vi "Shift Zero (single).vi"(8 "error in (no error)":errorcluster, 10 "Zero x index":i32, 11 "XY-data":cluster{"X-array":dbl[], "Y-array":dbl[]}) -> (0 "error out":errorcluster, 3 "Shifted XY-data out":cluster{"X-array":dbl[], "Y-array":dbl[]} {"Y-array" format="%.2p"; "X-array" format="%.2p"})   [LabVIEW 2016, in "xy_utilities.lvlib"]
doc: "Shift the zero value of the x array by giving a new fractional x index.\n\nWire data to the data input to determine the polymorphic instance to use or manually select the instance."
uses:
  xy_utilities.lvlib
  Sort (single).vi
  <vilib>/gmath/NI_Gmath.lvlib
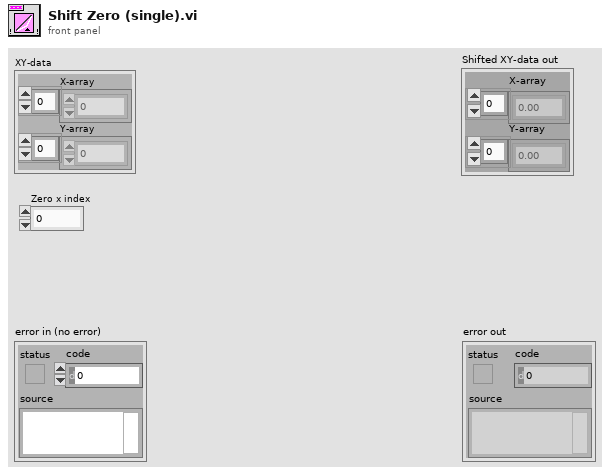
[diagram p1: front panel]
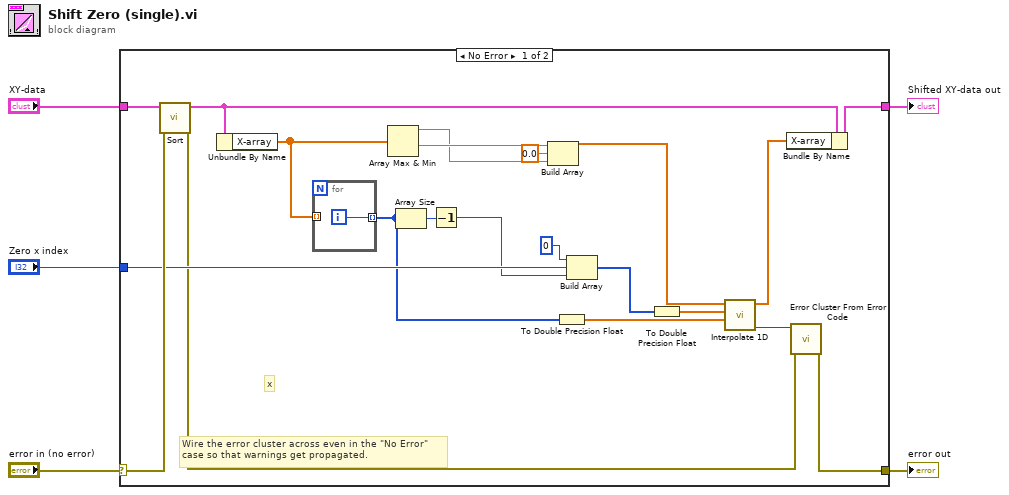
[diagram p0: block diagram]
diagram:
  n1 = case shown="No Error" "error in (no error)" {
    selector: "error in (no error)" -> [w20 w29]
    tunnel: [w8 w29] -> w4
    tunnel: "XY-data" -> [w11 w28]
    tunnel: [w26 w28] -> w2
    tunnel: "Zero x index" -> [w17 _]
    frame No Error {
      # "x"
      # "Wire the error cluster across even in the \"No Error\"\ncase so that warnings get propagated."
      n2 = call-poly "Sort.vi"("error in (no error)"=w20, "XY-data"=w11) -> ("error out"=w9:errorcluster, "Sorted XY-data out"=w10:cluster{"X-array":dbl[], "Y-array":dbl[]})  [unwired: 8 in]
      n3 = Unbundle By Name(w10) -> ("X-array"=w12:dbl[])
      n4 = for {
        tunnel: w12 -> [_] mode=indexing
        tunnel: [w27] -> w13 mode=indexing
        i -> [w27]
      }
      n5 = Array Max & Min(array=w12) -> (max value=w22:dbl, min value=w23:dbl)  [unwired: 2 out]
      n6 = Array Size(array=w13) -> (size(s)=w18:i32)
      n7 = Decrement(x=w18) -> (x-1=w16:i32)
      n8 = Build Array(w23, 0.0 ("element"), w22) -> (w14:dbl[])
      n9 = To Double Precision Float(number=w13) -> (double precision float=w6:dbl[])
      n10 = Build Array(0 ("element"), w17, w16) -> (w15:i32[])
      n11 = To Double Precision Float(number=w15) -> (double precision float=w7:dbl[])
      n12 = call <vilib>:"Interpolate 1D.vi"("xi"=w6, "X"=w7, "Y"=w14) -> ("error"=w25:i32, "yi"=w24:dbl[])  [unwired: 6 in, 1 out]
      n13 = Bundle By Name(cluster=w10, "X-array"=w24) -> (w26:cluster{"X-array":dbl[], "Y-array":dbl[]})
      n14 = call <vilib>:"Error Cluster From Error Code.vi"("error in (no error)"=w9, "error code (0)"=w25) -> ("error out"=w8:errorcluster)  [unwired: 7 in]
    }
    frame Error {
    }
  }
  "error out" <- w4
  "Shifted XY-data out" <- w2
